vi "Init.vi"(6 "Export Data Locations":string[](array[string]), 8 "error in (no error)":errorcluster, 9 "Span":string, 10 "Measurement Name":string, 11 "Standard":string) -> (0 "error out":errorcluster, 3 "Harmonics_Relative_Power out":refnum<class "RxBN dBmHz Calculation.lvclass">)   [LabVIEW 2016, in "SeqAuto Evaluations.lvlib" / "RxBN dBmHz Calculation.lvclass"]
uses:
  RxBN dBmHz Calculation.lvclass
  C:/Projects/STS/Common/Sequence Automation/Plugins/SeqAuto IEvaluation.lvlibp/SeqAuto IEvaluation.lvclass
  RxBN dBmHz Calculation.lvclass/RxBN dBmHz Calculation.ctl
  Write Export Data Locations.vi
  Write Span.vi
  Plugins/SeqAuto IEvaluation.lvlibp/Write Measurement Name.vi
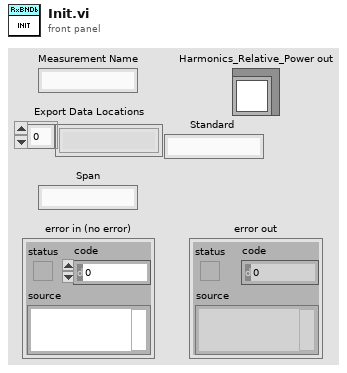
[diagram p1: front panel]
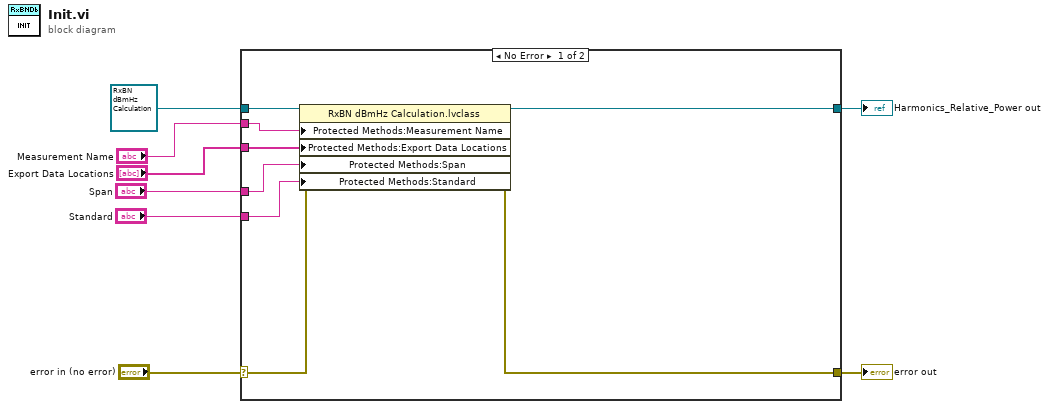
[diagram p0: block diagram]
diagram:
  n1 = case shown="No Error" "error in (no error)" {
    selector: "error in (no error)" -> [w16 w18]
    tunnel: [w15 w18] -> w7
    tunnel: [w13 w17] -> w5
    tunnel: refnum<class "RxBN dBmHz Calculation.lvclass"> refnum ("Harmonics_Relative_Power in") -> [w14 w17]
    tunnel: "Measurement Name" -> [w12 _]
    tunnel: "Export Data Locations" -> [w11 _]
    tunnel: "Span" -> [w10 _]
    tunnel: "Standard" -> [w9 _]
    frame No Error {
      n2 = property class="RxBN dBmHz Calculation.lvclass"(reference=w14, error in=w16, "Protected Methods:Measurement Name"=w12, "Protected Methods:Export Data Locations"=w11, "Protected Methods:Span"=w10, "Protected Methods:Standard"=w9) -> (reference out=w13:refnum<class "RxBN dBmHz Calculation.lvclass">, error out=w15:errorcluster)
    }
    frame Error {
    }
  }
  "error out" <- w7
  "Harmonics_Relative_Power out" <- w5
